vi "Teleop.vi"(10 "Match Info":T3={"Autonomous Elapsed Seconds"=0.0, "TeleOp Elapsed Seconds"=7.179, "Disabled Elapsed Seconds"=0.0, "Visited Autonomous"=FALSE, "Visited TeleOp"=TRUE, "Visited Disabled"=FALSE, "Autonomous Settings"={"Autonomous Style"=enum."Independent", "VI Refnum"=refnum}}, 11 "Call Context":T4=enum."Stop") -> ()   [LabVIEW 2020]
doc: "This VI is called for each TeleOp packet received from the DS where the robot is not disabled. It is often used to read from the joysticks and update I/O or to update setpoints for timed control loops. It should complete and return within 20 milliseconds or it may miss DS packets."
uses:
  <vilib>/Rock Robotics/WPI/DriverStation/WPI_DriverStationDerivedRobotMode.ctl
  <vilib>/Rock Robotics/WPI/DriverStation/WPI_DriverStationMatch Info.ctl
  <vilib>/Rock Robotics/WPI/ThirdParty/REV Robotics/REVLib/Typedef/Spark MAX Control Type.ctl
  <vilib>/Rock Robotics/WPI/ThirdParty/Sensors/navX/_TypeDefs/FRIC_navX_DeviceNumbersTypeDef.ctl
  <vilib>/Rock Robotics/WPI/ThirdParty/Phoenix-LabVIEW/CANCoder/Get/CTRE_Phoenix_CANcoder_GetSensorData.vi
  <vilib>/Rock Robotics/WPI/Utilities/WPI_GetSetVariantRefNum.vi
  <vilib>/addons/control/pid/pid.llb/PID (DBL).vi
  Robot Global Data.vi
  <vilib>/addons/control/pid/NI_PID_pid.lvlib
panel:
  in  "target angle":dbl=180.0
  out "Displacement":T1={"Velocity X"=0.000396728515625, "Velocity Y"=0.0001678466796875, "Velocity Z"=0.0062255859375, "Displacement X"=-3.0426025390625, "Displacement Y"=-16.154144287109375, "Displacement Z"=197.558837890625}
  out "MPUTemp":dbl=33.66
  in  "dt (s)":dbl=-1.0 format="%.3f"
  out "Yaw":dbl=-4.92
  in  "ScaleSpeed":dbl=0.5
  in  "PID gains 2":T2={"proportional gain (Kc)"=0.004667, "integral time (Ti, min)"=0.0, "derivative time (Td, min)"=0.0} {"derivative time (Td, min)" format="%.10f"; "integral time (Ti, min)" format="%.10f"; "proportional gain (Kc)" format="%.10f"}
  # "NOW WITH 200% MORE REV!!!!"
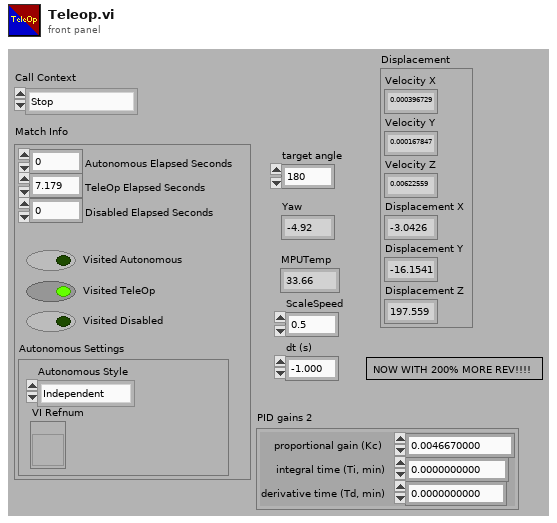
[diagram p1: front panel]
types:
  T1 = cluster{"Velocity X":dbl, "Velocity Y":dbl, "Velocity Z":dbl, "Displacement X":dbl, "Displacement Y":dbl, "Displacement Z":dbl}
  T2 = cluster{"proportional gain (Kc)":dbl, "integral time (Ti, min)":dbl, "derivative time (Td, min)":dbl}
  T3 = typedef "WPI_DriverStationMatch Info.ctl" = cluster{"Autonomous Elapsed Seconds":dbl, "TeleOp Elapsed Seconds":dbl, "Disabled Elapsed Seconds":dbl, "Visited Autonomous":bool, "Visited TeleOp":bool, "Visited Disabled":bool, "Autonomous Settings":cluster{"Autonomous Style":enum16{"Iterative", "Independent"}, "VI Refnum":refnum<vi>}}
  T4 = typedef "WPI_DriverStationDerivedRobotMode.ctl" = enum16{"Init", "Execute", "Stop"}
  T5 = typedef "FRIC_navX_DeviceNumbersTypeDef.ctl" = enum16{"Dev0", "Dev1", "Dev2", "Dev3"}
  T6 = typedef "Spark MAX Control Type.ctl" = enum16{"Percent VBus", "Voltage", "Velocity", "Position", "Smart Motion", "Current", "Smart Velocity"}
  T7 = typedef "WPI_JoystickDevRef.ctl" = cluster{"Device":T8}
  T8 = typedef "WPI_JoystickDeviceEnum.ctl" = enum16{"USB 0", "USB 1", "USB 2", "USB 3", "USB 4", "USB 5"}
  T9 = cluster{"Yaw":dbl, "Roll":dbl, "Pitch":dbl, "Heading":dbl, "Fused Heading":dbl}
  T10 = typedef "CTRE_Phoenix_CANcoder_DeviceRef.ctl" = cluster{"DeviceStatus":errorcluster, "Device Number":u8, "Handle":u64, "UsageFrame":u32, "Library Path":path}
  T11 = typedef "WPI_MotorControlDeviceRef.ctl" = cluster{"DeviceStatus":errorcluster, "Type":T12, "PWM":cluster{"PWM Channel":T13, "DeadBand":T14}, "CAN":cluster{"Device Number":u8, "SetOutput VI Ref":variant, "GetOutput VI Ref":variant, "Enable VI Ref":variant, "Disable VI Ref":variant, "Data":variant}, "Invert":bool, "DIO PWM":cluster{"PWM \"Enable\" Channel":T13, "DIOChannel":T15, "PWM Rate":dbl}}
  T12 = typedef "WPI_MotorControlType.ctl" = enum16{"PWM", "CAN", "DIO PWM"}
  T13 = typedef "FPGA_DIOPWMChannel.ctl" = enum8{"PWM 0", "PWM 1", "PWM 2", "PWM 3", "PWM 4", "PWM 5", "PWM 6", "PWM 7", "PWM 8", "PWM 9", "PWM MXP 0", "PWM MXP 1", "PWM MXP 2", "PWM MXP 3", "PWM MXP 4", "PWM MXP 5", "PWM MXP 6", "PWM MXP 7", "PWM MXP 8", "PWM MXP 9", "Invalid"}
  T14 = typedef "WPI_PWMDeadband.ctl" = cluster{"Name":string, "maxPositivePwm":i32, "minPositivePwm":i32, "centerPwm":i32, "maxNegativePwm":i32, "minNegativePwm":i32, "angularRange":u16}
  T15 = typedef "FPGA_DIOChannel.ctl" = enum8{"DIO 0", "DIO 1", "DIO 2", "DIO 3", "DIO 4", "DIO 5", "DIO 6", "DIO 7", "DIO 8", "DIO 9", "DIO MXP 0", "DIO MXP 1", "DIO MXP 2", "DIO MXP 3", "DIO MXP 4", "DIO MXP 5", "DIO MXP 6", "DIO MXP 7", "DIO MXP 8", "DIO MXP 9", "DIO MXP 10", "DIO MXP 11", "DIO MXP 12", "DIO MXP 13", "DIO MXP 14", "DIO MXP 15", "SPI Port CS1", "SPI Port CS2", "SPI Port CS3", "SPI Port MISO", "SPI Port MOSI", "Invalid"}
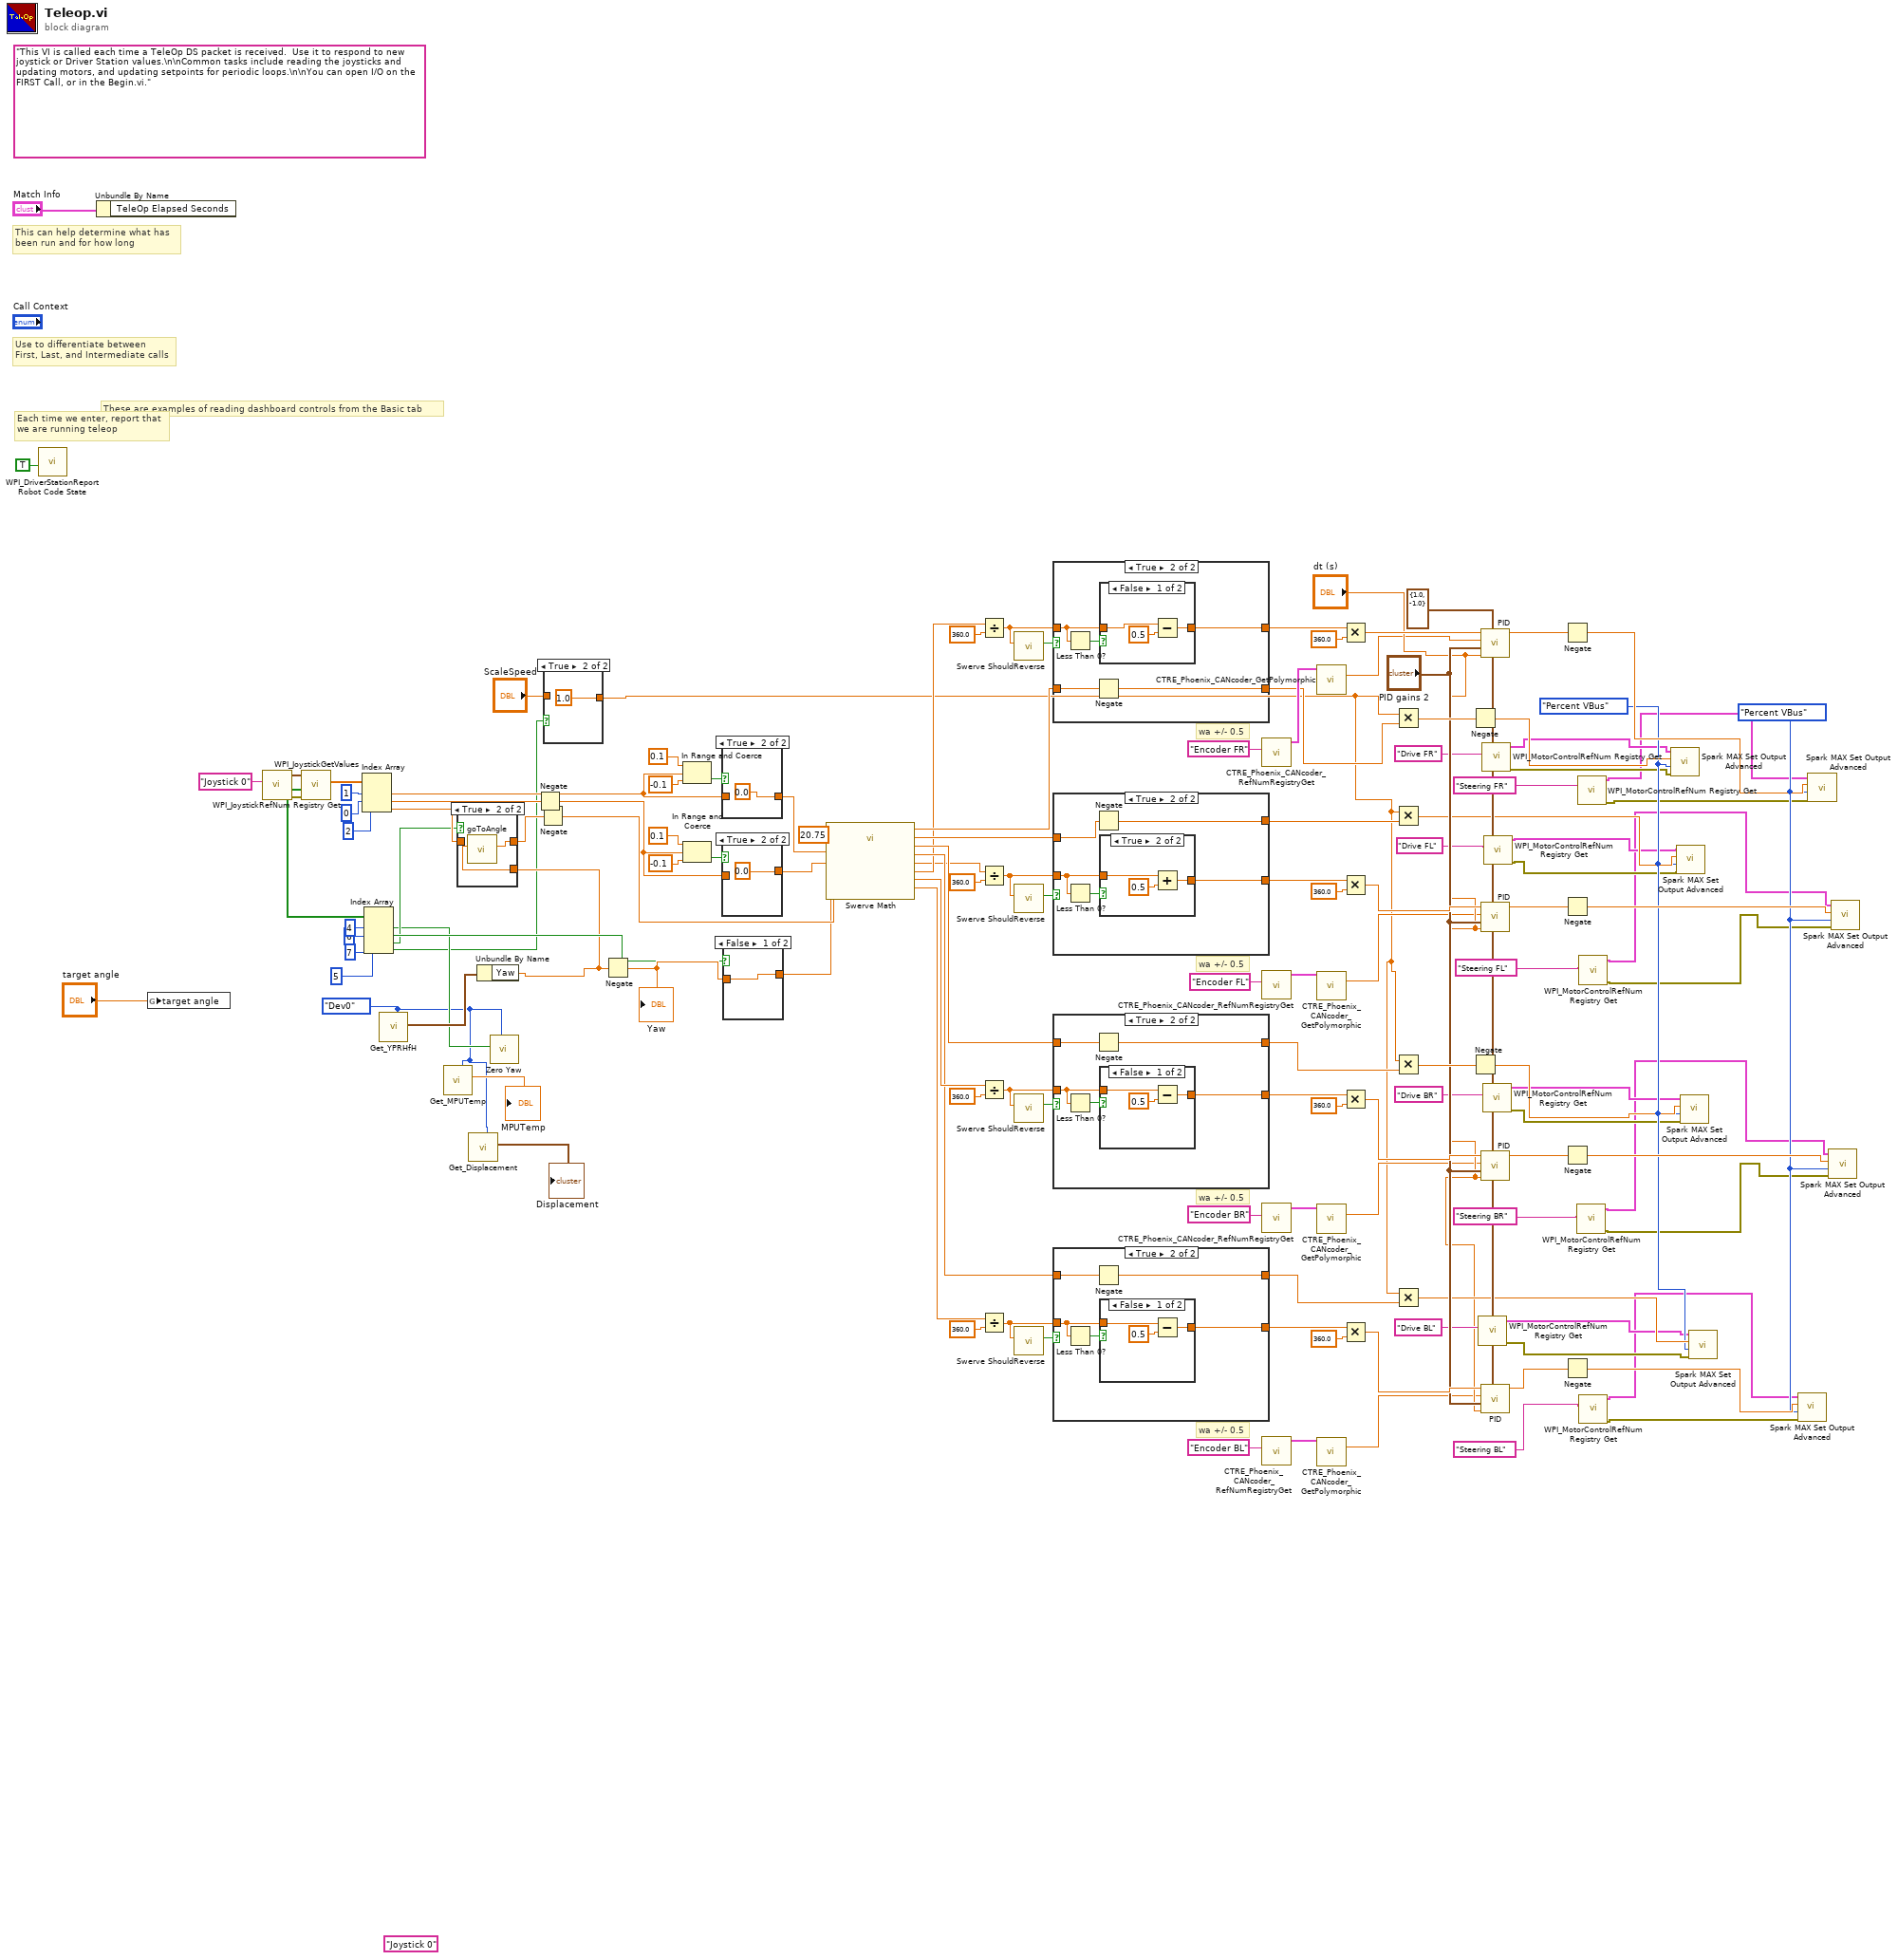
[diagram p0: block diagram]
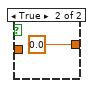
[diagram p4: hidden frame]
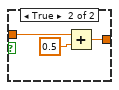
[diagram p6: hidden frame]
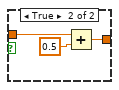
[diagram p8: hidden frame]
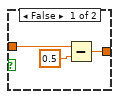
[diagram p10: hidden frame]
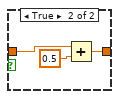
[diagram p12: hidden frame]
diagram:
  w7 = FRIC_navX_DeviceNumbersTypeDef."Dev0" ("Device Number")
  w57 = Spark_MAX_Control_Type."Percent VBus" ("Control Mode")
  w62 = Spark_MAX_Control_Type."Percent VBus" ("Control Mode")
  (unwired) "Joystick 0" ("refnum name")
  w67 = cluster{"output high":dbl, "output low":dbl} {"output high"=1.0, "output low"=-1.0} ("output range")
  w132 = 20.75 ("Trackwidth (W)")
  (unwired) "This VI is called each time a TeleOp DS packet is received.  Use it to respond to new joystick or Driver Station values.\n\nCommon tasks include reading the joysticks and updating motors, and updating setpoints for periodic loops.\n\nYou can open I/O on the FIRST Call, or in the Begin.vi."
  # "wa +/- 0.5"
  # "wa +/- 0.5"
  # "wa +/- 0.5"
  # "wa +/- 0.5"
  # "These are examples of reading dashboard controls from the Basic tab"
  # "Each time we enter, report that\nwe are running teleop"
  # "Use to differentiate between\nFirst, Last, and Intermediate calls"
  # "This can help determine what has\nbeen run and for how long"
  n1 = call <vilib>:"WPI_DriverStationReport Robot Code State.vi"("TeleOp"=TRUE ("Autonomous")) -> ()  [unwired: 10 in, 1 out]
  n2 = Unbundle By Name("Match Info") -> ()  [unwired: 1 out]
  n3 = global write "Robot Global Data.vi" "target angle"("target angle") -> ()
  n4 = call <vilib>:"WPI_JoystickRefNum Registry Get.vi"("refnum name"="Joystick 0") -> ("error out"=w128:errorcluster, "JoystickDevRef"=w127:T7)  [unwired: 9 in]
  n5 = call <vilib>:"WPI_JoystickGetValues.vi"("error in (no error)"=w128, "JoystickDevRef"=w127) -> ("Buttons"=w23:bool[], "Axes"=w125:dbl[])  [unwired: 5 in, 3 out]
  n6 = Index Array(array=w125, index #1=1 ("index"), index #2=0 ("index"), index #3=2 ("index")) -> (element #1=w116:dbl, element #2=w26:dbl, element #3=w12:dbl)
  n7 = Index Array(array=w23, index #1=4 ("index"), index #2=6 ("index"), index #3=7 ("index"), index #4=5 ("index")) -> (element #1=w9:bool, element #2=w17:bool, element #3=w11:bool, element #4=w2:bool)
  n8 = call <vilib>:"Get_YPRHfH.vi"("Device Number"=w7) -> ("YRPHfH"=w20:T9)  [unwired: 10 in]
  n9 = call <vilib>:"Get_MPUTemp.vi"("Device Number"=w7) -> ("MPUTemp"=→"MPUTemp":dbl)  [unwired: 10 in]
  n10 = call <vilib>:"Get_Displacement.vi"("Device Number"=w7) -> ("Displacement"=→"Displacement":T1)  [unwired: 10 in]
  n11 = Unbundle By Name(w20) -> ("Yaw"=w10:dbl)
  n12 = case shown="True" w11 {
    tunnel: [w135 w137] -> w13
    tunnel: w12 -> [w135 _]
    tunnel: w10 -> [_ w136]
    frame False {
    }
    frame True {
      n13 = call "goToAngle.vi"("gyro"=w136) -> ("x2"=w137:dbl)  [unwired: 10 in]
    }
  }
  n14 = call <vilib>:"Zero Yaw.vi"("Device Number"=w7, "Zero"=w9) -> ()  [unwired: 10 in]
  n15 = Negate(x=w26) -> (-x=w25:dbl)
  n16 = Negate(x=w13) -> (-x=w24:dbl)
  n17 = case shown="True" w2 {
    tunnel: [w138 1.0 ("upper limit")] -> w4
    tunnel: "ScaleSpeed" -> [w138 _]
    frame False {
    }
    frame True {
    }
  }
  n18 = Negate(x=w10) -> (-x=w18:dbl)
  "Yaw" <- w18
  n19 = In Range and Coerce(upper limit=0.1, x=w116, lower limit=-0.1) -> (In Range?=w120:bool)  [unwired: 1 out]
  n20 = In Range and Coerce(upper limit=0.1, x=w25, lower limit=-0.1) -> (In Range?=w119:bool)  [unwired: 1 out]
  n21 = case shown="True" w120 {
    tunnel: [w140 0.0 ("upper limit")] -> w114
    tunnel: w116 -> [w140 _]
    frame False {
    }
    frame True {
    }
  }
  n22 = case shown="True" w119 {
    tunnel: [w142 0.0 ("upper limit")] -> w115
    tunnel: w25 -> [w142 _]
    frame False {
    }
    frame True {
    }
  }
  n23 = case shown="False" w17 {
    tunnel: [w144 0.0 ("upper limit")] -> w19
    tunnel: w18 -> [w144 _]
    frame False {
    }
    frame True {
    }
  }
  n24 = call "Swerve Math.vi"("Trackwidth (W)"=w132, "Wheelbase (L)"=w132, "Y -FWD"=w114, "X1 STR"=w115, "X2 RCW"=w24, "Gyro Angle in degrees"=w19) -> ("wa3"=w71:dbl, "wa4"=w69:dbl, "ws1"=w74:dbl, "ws2"=w73:dbl, "ws3"=w72:dbl, "ws4"=w70:dbl, "wa2"=w16:dbl, "wa1"=w15:dbl)  [unwired: 2 in]
  n25 = Divide(x=w16, y=360.0) -> (x/y=w111:dbl)
  n26 = Divide(x=w15, y=360.0) -> (x/y=w100:dbl)
  n27 = Divide(x=w71, y=360.0) -> (x/y=w90:dbl)
  n28 = Divide(x=w69, y=360.0) -> (x/y=w79:dbl)
  n29 = call "Swerve ShouldReverse.vi"("wa in"=w111) -> ("shouldReverse out"=w112:bool)  [unwired: 10 in]
  n30 = call "Swerve ShouldReverse.vi"("wa in"=w100) -> ("shouldReverse out"=w101:bool)  [unwired: 10 in]
  n31 = call "Swerve ShouldReverse.vi"("wa in"=w90) -> ("shouldReverse out"=w91:bool)  [unwired: 10 in]
  n32 = call "Swerve ShouldReverse.vi"("wa in"=w79) -> ("shouldReverse out"=w80:bool)  [unwired: 10 in]
  n33 = case shown="True" w112 {
    tunnel: w74 -> [w147 w148]
    tunnel: w111 -> [w146 w151]
    tunnel: [w147 w149] -> w110
    tunnel: [w146 w150] -> w109
    frame False {
    }
    frame True {
      n34 = Less Than 0?(x=w151) -> (x < 0?=w152:bool)
      n35 = Negate(x=w148) -> (-x=w149:dbl)
      n36 = case shown="False" w152 {
        tunnel: w151 -> [w154 w157]
        tunnel: [w153 w156] -> w150
        frame False {
          n37 = Subtract(x=w154, y=0.5) -> (x-y=w153:dbl)
        }
        frame True {
          n38 = Add(x=w157, y=0.5) -> (x+y=w156:dbl)
        }
      }
    }
  }
  n39 = case shown="True" w101 {
    tunnel: w73 -> [w160 w161]
    tunnel: w100 -> [w159 w164]
    tunnel: [w160 w162] -> w99
    tunnel: [w159 w163] -> w98
    frame False {
    }
    frame True {
      n40 = Less Than 0?(x=w164) -> (x < 0?=w165:bool)
      n41 = Negate(x=w161) -> (-x=w162:dbl)
      n42 = case shown="True" w165 {
        tunnel: w164 -> [w167 w170]
        tunnel: [w166 w169] -> w163
        frame False {
          n43 = Subtract(x=w167, y=0.5) -> (x-y=w166:dbl)
        }
        frame True {
          n44 = Add(x=w170, y=0.5) -> (x+y=w169:dbl)
        }
      }
    }
  }
  n45 = case shown="True" w91 {
    tunnel: w72 -> [w173 w174]
    tunnel: w90 -> [w172 w177]
    tunnel: [w173 w175] -> w89
    tunnel: [w172 w176] -> w88
    frame False {
    }
    frame True {
      n46 = Less Than 0?(x=w177) -> (x < 0?=w178:bool)
      n47 = Negate(x=w174) -> (-x=w175:dbl)
      n48 = case shown="False" w178 {
        tunnel: w177 -> [w180 w183]
        tunnel: [w179 w182] -> w176
        frame False {
          n49 = Subtract(x=w180, y=0.5) -> (x-y=w179:dbl)
        }
        frame True {
          n50 = Add(x=w183, y=0.5) -> (x+y=w182:dbl)
        }
      }
    }
  }
  n51 = case shown="True" w80 {
    tunnel: w70 -> [w186 w187]
    tunnel: w79 -> [w185 w190]
    tunnel: [w186 w188] -> w78
    tunnel: [w185 w189] -> w77
    frame False {
    }
    frame True {
      n52 = Less Than 0?(x=w190) -> (x < 0?=w191:bool)
      n53 = Negate(x=w187) -> (-x=w188:dbl)
      n54 = case shown="False" w191 {
        tunnel: w190 -> [w193 w196]
        tunnel: [w192 w195] -> w189
        frame False {
          n55 = Subtract(x=w193, y=0.5) -> (x-y=w192:dbl)
        }
        frame True {
          n56 = Add(x=w196, y=0.5) -> (x+y=w195:dbl)
        }
      }
    }
  }
  n57 = call <vilib>:"CTRE_Phoenix_CANcoder_RefNumRegistryGet.vi"("refnum name"="Encoder FR") -> ("CTRE_CANcoder_DeviceRef"=w130:T10)  [unwired: 9 in, 1 out]
  n58 = call <vilib>:"CTRE_Phoenix_CANcoder_RefNumRegistryGet.vi"("refnum name"="Encoder FL") -> ("CTRE_CANcoder_DeviceRef"=w104:T10)  [unwired: 9 in, 1 out]
  n59 = call <vilib>:"CTRE_Phoenix_CANcoder_RefNumRegistryGet.vi"("refnum name"="Encoder BR") -> ("CTRE_CANcoder_DeviceRef"=w94:T10)  [unwired: 9 in, 1 out]
  n60 = call <vilib>:"CTRE_Phoenix_CANcoder_RefNumRegistryGet.vi"("refnum name"="Encoder BL") -> ("CTRE_CANcoder_DeviceRef"=w83:T10)  [unwired: 9 in, 1 out]
  n61 = call-poly <vilib>:"CTRE_Phoenix_CANcoder_GetPolymorphic.vi"("CTRE_CANcoder_DeviceRef"=w130) -> ("Position"=w28:dbl)  [unwired: 10 in, 4 out]
  n62 = call-poly <vilib>:"CTRE_Phoenix_CANcoder_GetPolymorphic.vi"("CTRE_CANcoder_DeviceRef"=w104) -> ("Position"=w29:dbl)  [unwired: 10 in, 4 out]
  n63 = call-poly <vilib>:"CTRE_Phoenix_CANcoder_GetPolymorphic.vi"("CTRE_CANcoder_DeviceRef"=w94) -> ("Position"=w30:dbl)  [unwired: 10 in, 4 out]
  n64 = call-poly <vilib>:"CTRE_Phoenix_CANcoder_GetPolymorphic.vi"("CTRE_CANcoder_DeviceRef"=w83) -> ("Position"=w27:dbl)  [unwired: 10 in, 4 out]
  n65 = Multiply(x=w109, y=360.0) -> (x*y=w108:dbl)
  n66 = Multiply(x=w98, y=360.0) -> (x*y=w97:dbl)
  n67 = Multiply(x=w88, y=360.0) -> (x*y=w87:dbl)
  n68 = Multiply(x=w77, y=360.0) -> (x*y=w76:dbl)
  n69 = Multiply(x=w4, y=w110) -> (x*y=w106:dbl)
  n70 = Multiply(x=w4, y=w99) -> (x*y=w60:dbl)
  n71 = Multiply(x=w4, y=w89) -> (x*y=w85:dbl)
  n72 = Multiply(x=w4, y=w78) -> (x*y=w58:dbl)
  n73 = Negate(x=w106) -> (-x=w61:dbl)
  n74 = Negate(x=w85) -> (-x=w59:dbl)
  n75 = call <vilib>:"WPI_MotorControlRefNum Registry Get.vi"("refnum name"="Drive BL") -> ("error out"=w37:errorcluster, "MotorControlDevRef"=w38:T11)  [unwired: 9 in]
  n76 = call-poly <vilib>:"PID.vi"("output range"=w67, "dt (s)"="dt (s)", "PID gains"="PID gains 2", "process variable"=w28, "setpoint"=w108) -> ("output"=w131:dbl)  [unwired: 5 in, 1 out]
  n77 = call-poly <vilib>:"PID.vi"("output range"=w67, "dt (s)"="dt (s)", "PID gains"="PID gains 2", "process variable"=w29, "setpoint"=w97) -> ("output"=w105:dbl)  [unwired: 5 in, 1 out]
  n78 = call-poly <vilib>:"PID.vi"("output range"=w67, "dt (s)"="dt (s)", "PID gains"="PID gains 2", "process variable"=w30, "setpoint"=w87) -> ("output"=w95:dbl)  [unwired: 5 in, 1 out]
  n79 = call-poly <vilib>:"PID.vi"("output range"=w67, "dt (s)"="dt (s)", "PID gains"="PID gains 2", "process variable"=w27, "setpoint"=w76) -> ("output"=w84:dbl)  [unwired: 5 in, 1 out]
  n80 = call <vilib>:"WPI_MotorControlRefNum Registry Get.vi"("refnum name"="Drive FR") -> ("error out"=w54:errorcluster, "MotorControlDevRef"=w55:T11)  [unwired: 9 in]
  n81 = call <vilib>:"WPI_MotorControlRefNum Registry Get.vi"("refnum name"="Drive BR") -> ("error out"=w42:errorcluster, "MotorControlDevRef"=w43:T11)  [unwired: 9 in]
  n82 = call <vilib>:"WPI_MotorControlRefNum Registry Get.vi"("refnum name"="Drive FL") -> ("error out"=w48:errorcluster, "MotorControlDevRef"=w49:T11)  [unwired: 9 in]
  n83 = Negate(x=w131) -> (-x=w66:dbl)
  n84 = Negate(x=w105) -> (-x=w65:dbl)
  n85 = Negate(x=w95) -> (-x=w64:dbl)
  n86 = Negate(x=w84) -> (-x=w63:dbl)
  n87 = call <vilib>:"WPI_MotorControlRefNum Registry Get.vi"("refnum name"="Steering BR") -> ("error out"=w40:errorcluster, "MotorControlDevRef"=w41:T11)  [unwired: 9 in]
  n88 = call <vilib>:"WPI_MotorControlRefNum Registry Get.vi"("refnum name"="Steering FR") -> ("error out"=w51:errorcluster, "MotorControlDevRef"=w52:T11)  [unwired: 9 in]
  n89 = call <vilib>:"WPI_MotorControlRefNum Registry Get.vi"("refnum name"="Steering FL") -> ("error out"=w45:errorcluster, "MotorControlDevRef"=w46:T11)  [unwired: 9 in]
  n90 = call <vilib>:"WPI_MotorControlRefNum Registry Get.vi"("refnum name"="Steering BL") -> ("error out"=w34:errorcluster, "MotorControlDevRef"=w35:T11)  [unwired: 9 in]
  n91 = call <vilib>:"Spark MAX Set Output Advanced.vi"("error in (no error)"=w54, "Control Mode"=w57, "Setpoint"=w61, "MotorControlDevRef"=w55) -> ()  [unwired: 6 in, 2 out]
  n92 = call <vilib>:"Spark MAX Set Output Advanced.vi"("error in (no error)"=w48, "Control Mode"=w57, "Setpoint"=w60, "MotorControlDevRef"=w49) -> ()  [unwired: 6 in, 2 out]
  n93 = call <vilib>:"Spark MAX Set Output Advanced.vi"("error in (no error)"=w42, "Control Mode"=w57, "Setpoint"=w59, "MotorControlDevRef"=w43) -> ()  [unwired: 6 in, 2 out]
  n94 = call <vilib>:"Spark MAX Set Output Advanced.vi"("error in (no error)"=w37, "Control Mode"=w57, "Setpoint"=w58, "MotorControlDevRef"=w38) -> ()  [unwired: 6 in, 2 out]
  n95 = call <vilib>:"Spark MAX Set Output Advanced.vi"("error in (no error)"=w34, "Control Mode"=w62, "Setpoint"=w63, "MotorControlDevRef"=w35) -> ()  [unwired: 6 in, 2 out]
  n96 = call <vilib>:"Spark MAX Set Output Advanced.vi"("error in (no error)"=w51, "Control Mode"=w62, "Setpoint"=w66, "MotorControlDevRef"=w52) -> ()  [unwired: 6 in, 2 out]
  n97 = call <vilib>:"Spark MAX Set Output Advanced.vi"("error in (no error)"=w40, "Control Mode"=w62, "Setpoint"=w64, "MotorControlDevRef"=w41) -> ()  [unwired: 6 in, 2 out]
  n98 = call <vilib>:"Spark MAX Set Output Advanced.vi"("error in (no error)"=w45, "Control Mode"=w62, "Setpoint"=w65, "MotorControlDevRef"=w46) -> ()  [unwired: 6 in, 2 out]
